vi "dfd_Arc Elliptic Tangent.vi"(2 "k'":dbl=1.0 format="%.2f", 3 "u":dbl=1.0 format="%.2f") -> (0 "convergence":bool=TRUE, 1 "arcsc(u,k)":dbl format="%.6f")   [LabVIEW 2017, in "NI_DigFilter_Design.lvlib"]
uses:
  <vilib>/addons/Digital Filter Design/NI_DigFilter_Design.lvlib
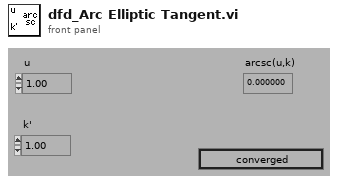
[diagram p1: front panel]
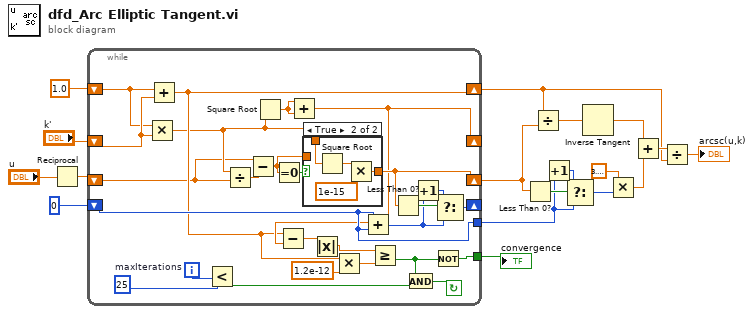
[diagram p0: block diagram]
diagram:
  n1 = Reciprocal(x="u") -> (1/x=w15:dbl)
  n2 = while {
    tunnel: [w28] -> w10
    tunnel: [w34] -> w13
    shift-left: 0 -> [w28]
    shift-right: [w31] -> _
    shift-left: w15 -> [w21]
    shift-right: [w33] -> w9
    shift-left: "k'" -> [w27]
    shift-right: [w25] -> _
    shift-left: 1.0 -> [w24]
    shift-right: [w23] -> w2
    i -> [w44]
    stop <- w42 continue-if-true
    w41 = 25  # maxIterations
    n3 = Multiply(x=w24, y=w27) -> (x*y=w22:dbl)
    n4 = Add(x=w24, y=w27) -> (x+y=w23:dbl)
    n5 = Less?(x=w44, y=w41) -> (x < y?=w43:bool)
    n6 = Divide(x=w22, y=w21) -> (x/y=w20:dbl)
    n7 = Subtract(x=w21, y=w20) -> (x-y=w19:dbl)
    n8 = Square Root(x=w22) -> (sqrt(x)=w26:dbl)
    n9 = Equal To 0?(x=w19) -> (x = 0?=w40:bool)
    n10 = Add(x=w26, y=w26) -> (x+y=w25:dbl)
    n11 = Subtract(x=w23, y=w25) -> (x-y=w38:dbl)
    n12 = case shown="True" w40 {
      tunnel: w22 -> [_ w47]
      tunnel: [w45 w46] -> w33
      tunnel: w19 -> [w45 _]
      frame False {
      }
      frame True {
        n13 = Square Root(x=w47) -> (sqrt(x)=w48:dbl)
        n14 = Multiply(x=w48, y=1e-15) -> (x*y=w46:dbl)
      }
    }
    n15 = Absolute Value(x=w38) -> (abs(x)=w37:dbl)
    n16 = Multiply(x=w23, y=1.2e-12) -> (x*y=w36:dbl)
    n17 = Add(x=w28, y=w28) -> (x+y=w29:i32)
    n18 = Greater Or Equal?(x=w37, y=w36) -> (x >= y?=w35:bool)
    n19 = Less Than 0?(x=w33) -> (x < 0?=w32:bool)
    n20 = And(x=w35, y=w43) -> (x .and. y?=w42:bool)
    n21 = Increment(x=w29) -> (x+1=w30:i32)
    n22 = Not(x=w35) -> (.not. x?=w34:bool)
    n23 = Select(t=w30, s=w32, f=w29) -> (s? t:f=w31:i32)
  }
  "convergence" <- w13
  n24 = Less Than 0?(x=w9) -> (x < 0?=w11:bool)
  n25 = Divide(x=w2, y=w9) -> (x/y=w8:dbl)
  n26 = Increment(x=w10) -> (x+1=w12:i32)
  n27 = Select(t=w12, s=w11, f=w10) -> (s? t:f=w6:i32)
  n28 = Inverse Tangent(1:w8) -> (0:w5:dbl)
  n29 = Multiply(x=3.141592653589793, y=w6) -> (x*y=w4:dbl)
  n30 = Add(x=w5, y=w4) -> (x+y=w3:dbl)
  n31 = Divide(x=w3, y=w2) -> (x/y=→"arcsc(u,k)":dbl)
